vi "Template VI.vi"(8 "error in (no error)":errorcluster, 11 "Mock In":refnum<class "Mock.lvclass">) -> (0 "error out":errorcluster, 3 "Mock Out":refnum<class "Mock.lvclass">)   [LabVIEW 2020, in "Mock Class Generator.lvclass"]
uses:
  Mock Class Generator.lvclass
  Framework/Mock/Mock.lvclass
  Framework/Mock/Mock.lvclass/Mock.ctl
  Framework/VI Call/Create.vi
  Framework/Expectation/Expectation.lvclass
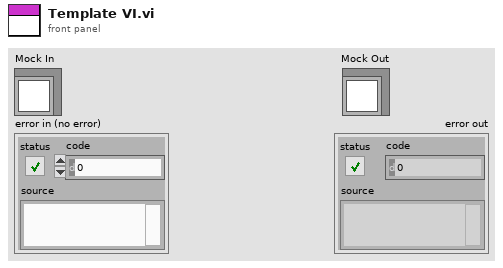
[diagram p1: front panel]
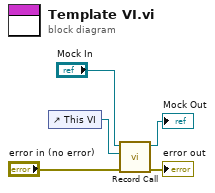
[diagram p0: block diagram]
diagram:
  n1 = control-ref of="This VI"() -> (w5:refnum<vi>)
  n2 = call "Record Call.vi"("error in (no error)"="error in (no error)", "This VI"=w5, "Mock In"="Mock In") -> ("error out"=→"error out":errorcluster, "Mock Out"=→"Mock Out":refnum<class "Mock.lvclass">)  [unwired: 7 in]
